vi "PythonNode_AddTwoDoubles.vi"() -> ()   [LabVIEW 2023]
doc: "This example demonstrates how to call a Python function and pass doubles as arguments. It uses a python function to compute the sum of two doubles."
uses:
  support/PythonVersionsEnum.ctl
panel:
  out "error out":errorcluster
  out "a + b":dbl
  in  "b":dbl=1.0
  in  "a":dbl=41.0
  in  "error in (no error)":errorcluster
  in  "Python version":T1
  # "Overview: Demonstrates how to call a Python function and pass doubles as arguments.\nRequirements: Python 3.6, 3.7, 3.8, 3.9 or 3.10 with the same bitness as LabVIEW.\nInstructions:\n1. Set the Python version to the version of Python you want to execute code in.\n2. Run the VI. You should see the result of adding \"a\" and \"b\" in the indicator \"a + b\".\n3. See comments on the block diagram of this VI and in \"ExamplePythonModule.py\" for more information about how the call python node passes arguments and handles return values."
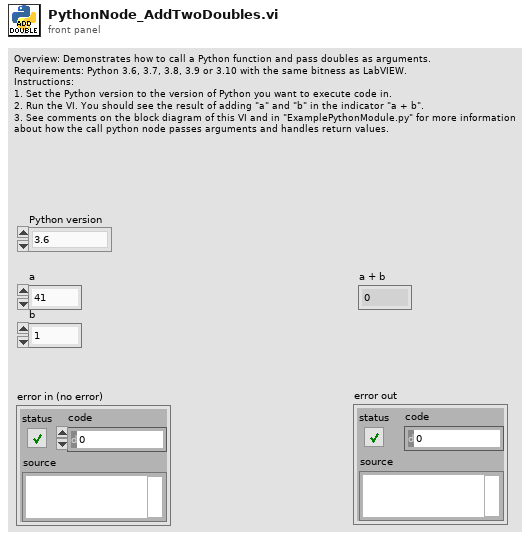
[diagram p1: front panel]
types:
  T1 = typedef "PythonVersionsEnum.ctl" = enum16{"3.6", "3.7", "3.8", "3.9", "3.10"}
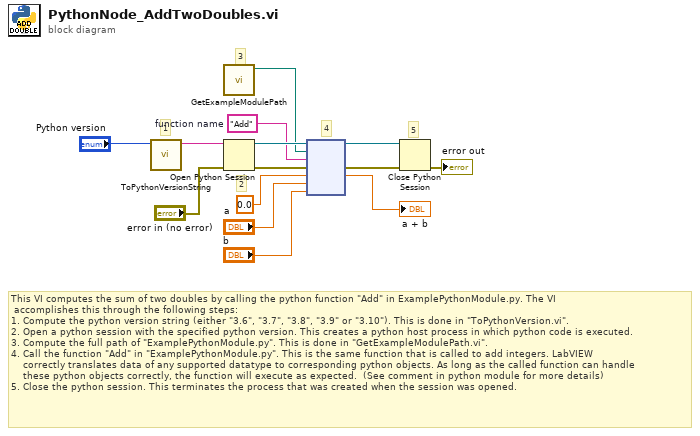
[diagram p0: block diagram]
diagram:
  w8 = "Add"  # function name
  # "5"
  # "4"
  # "2"
  # "3"
  # "1"
  # "This VI computes the sum of two doubles by calling the python function \"Add\" in ExamplePythonModule.py. The VI\n accomplishes this through the following steps:\n1. Compute the python version string (either \"3.6\", \"3.7\", \"3.8\", \"3.9\" or \"3.10\"). This is done in \"ToPythonVersion.vi\". \n2. Open a python session with the specified python version. This creates a python host process in which python code is executed.\n3. Compute the full path of \"ExamplePythonModule.py\". This is done in \"GetExampleModulePath.vi\".\n4. Call the function \"Add\" in \"ExamplePythonModule.py\". This is the same function that is called to add integers. LabVIEW \n    correctly translates data of any supported datatype to corresponding python objects. As long as the called function can handle\n    these python objects correctly, the function will execute as expected.  (See comment in python module for more details)\n5. Close the python session. This terminates the process that was created when the session was opened."
  n1 = call "ToPythonVersionString.vi"("python version"="Python version") -> ("python version string"=w14:string)  [unwired: 10 in]
  n2 = call "GetExampleModulePath.vi"() -> ("module path"=w9:path)  [unwired: 11 in]
  n3 = Open Python Session(python version=w14, 3:"error in (no error)") -> (session out=w11:refnum<k35>, error out=w10:errorcluster)  [unwired: 1 in]
  n4 = node(w11, w9, w8, w10, 0.0 ("a"), "a", "b") -> (w7:refnum<k35>, w6:errorcluster, →"a + b":dbl)  [unwired: 2 in, 2 out]
  n5 = Close Python Session(session in=w7, error in=w6) -> (11:→"error out":errorcluster)
